vi "RandomString.vi"(0 "Randomness":i32 caption="Randomness [bits]", 1 "Allowed characters":T1 caption="Allowed characters (Any)") -> (2 "Random string":string)   [LabVIEW 2017, in "GPString.lvlib"]
doc: "Creates a <B>Random string</B> of at least the specified <B>Randomness</B> (<B>Random string</B> is rounded up to a whole number of characters to cover the <B>Randomness</B> specification).\n\nThe optional <B>Allowed characters</B> lets you specify the character contents of the <B>Random string</B>, in case you have a use for the string which put limitations on which characters the string may contain (you may need the string for a folder name for instance). The following settings are available for <B>Allowed characters</B> (all char values are in decimal):\n\nAny (default): char values 0-255.\nAlphanumeric: char values 48-57 (numbers), 65-90 (upper case letters), and 97-122 (lower case letters).\nBinary: char values 48 and 49 (numbers 0 and 1).\nHexadecimal: char values 48-57 (numbers) and 65-70 (letters A-F).\nLetters: char values 65-90 (upper case letters) and 97-122 (lower case letters).\nLower case: char values 97-122 (lower case letters).\nNumbers: char values 48-57 (numbers).\nOctal: char values 48-55 (numbers 0-7).\nPrintable: char values 32-126.\nUpper case: char values 65-90 (upper case letters).\n\nThe reason <B>Randomness</B> is specified in number of bits instead of for example number of characters is that each character represents a variable number of random bits, depending on the <B>Allowed characters</B> setting. It gives a much more comprehendable value for randomness to specify the number of random bits than characters in that case.\n\nThis VI is inlined.\n\nSteen Schmidt\nGPower\n29/1 2013"
uses:
  GPString.lvlib
  Typedefs/AllowedChars.ctl
panel:
  # "Copyright © 2013\nSteen Schmidt, GPower\nSee enclosed license file for terms and conditions"
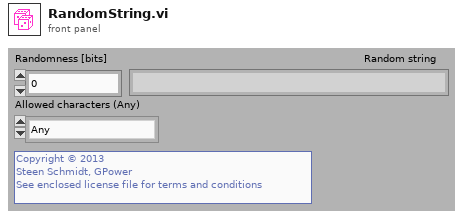
[diagram p1: front panel]
types:
  T1 = typedef "GPString.lvlib/AllowedChars.ctl" = enum16{"Any", "Alphanumeric", "Binary", "Hexadecimal", "Letters", "Lower case", "Numbers", "Octal", "Printable", "Upper case"}
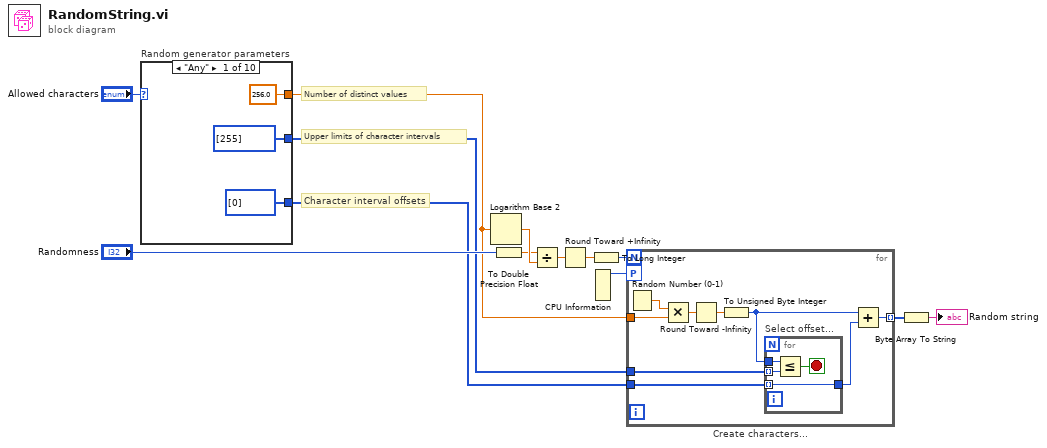
[diagram p0: block diagram]
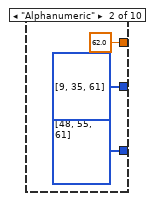
[diagram p2: hidden frame]
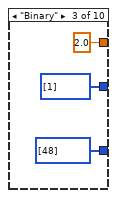
[diagram p3: hidden frame]
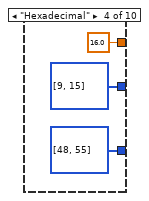
[diagram p4: hidden frame]
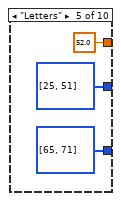
[diagram p5: hidden frame]
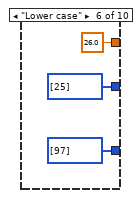
[diagram p6: hidden frame]
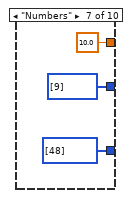
[diagram p7: hidden frame]
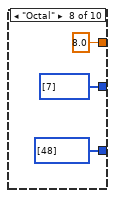
[diagram p8: hidden frame]
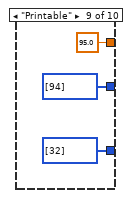
[diagram p9: hidden frame]
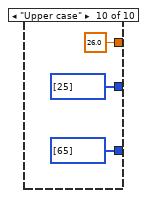
[diagram p10: hidden frame]
diagram:
  # "Character interval offsets"
  # "Upper limits of character intervals"
  # "Number of distinct values"
  n1 = case "Random generator parameters" shown="\"Any\"" "Allowed characters" {
    tunnel: [256.0 62.0 2.0 16.0 52.0 26.0 10.0 8.0 95.0 26.0] -> w6
    tunnel: [u8[] [255] u8[] [9, 35, 61] u8[] [1] u8[] [9, 15] u8[] [25, 51] u8[] [25] u8[] [9] u8[] [7] u8[] [94] u8[] [25]] -> w2
    tunnel: [u8[] [0] u8[] [48, 55, 61] u8[] [48] u8[] [48, 55] u8[] [65, 71] u8[] [97] u8[] [48] u8[] [48] u8[] [32] u8[] [65]] -> w1
    frame "Any" {
    }
    frame "Alphanumeric" {
    }
    frame "Binary" {
    }
    frame "Hexadecimal" {
    }
    frame "Letters" {
    }
    frame "Lower case" {
    }
    frame "Numbers" {
    }
    frame "Octal" {
    }
    frame "Printable" {
    }
    frame "Upper case" {
    }
  }
  n2 = Logarithm Base 2(1:w6) -> (0:w11:dbl)
  n3 = To Double Precision Float(number="Randomness") -> (double precision float=w5:dbl)
  n4 = Divide(x=w5, y=w11) -> (x/y=w10:dbl)
  n5 = Round Toward +Infinity(x=w10) -> (ceil(x): smallest int >= x=w9:dbl)
  n6 = CPU Information() -> (4:w7:i32)  [unwired: 3 out]
  n7 = To Long Integer(number=w9) -> (32bit integer=w8:i32)
  n8 = for "Create characters..." {
    N: w8 -> [_]
    workers-P: w7 -> [_]
    tunnel: w6 -> [w52]
    tunnel: w2 -> [w48]
    tunnel: w1 -> [w47]
    tunnel: [w45] -> w4 mode=indexing
    n9 = Random Number (0-1)() -> (number: 0 to 1=w51:dbl)
    n10 = Multiply(x=w51, y=w52) -> (x*y=w50:dbl)
    n11 = Round Toward -Infinity(1:w50) -> (0:w49:dbl)
    n12 = To Unsigned Byte Integer(number=w49) -> (unsigned 8bit integer=w44:u8)
    n13 = for "Select offset..." {
      tunnel: w48 -> [w55] mode=indexing
      tunnel: w44 -> [w56]
      tunnel: w47 -> [w53] mode=indexing
      tunnel: [w53] -> w46
      stop <- w54 stop-if-true
      n14 = Less Or Equal?(x=w56, y=w55) -> (x <= y?=w54:bool)
    }
    n15 = Add(x=w44, y=w46) -> (x+y=w45:u8)
  }
  n16 = Byte Array To String(unsigned byte array=w4) -> (string=→"Random string":string)
